vi "GV pockels main delay.vi"() -> ()   [LabVIEW 2017]
panel:
  out "PockelsMainDelay_tick":u32
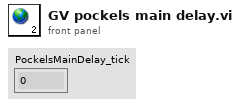
[diagram p1: front panel]
diagram:
